vi "Make.vi"(8 "error in (no error)":errorcluster, 9 "Item Refnum":refnum<vi>, 10 "Target":refnum<vi>, 11 "Abstract Message Rescripter":refnum<class "Abstract Message Rescripter.lvclass">) -> (0 "error out":errorcluster, 3 "Abstract Message Rescripter out":refnum<class "Abstract Message Rescripter.lvclass">)   [LabVIEW 2020, in "Message Rescripter.lvlib" / "Abstract Message Rescripter.lvclass"]
uses:
  Abstract Message Rescripter.lvclass
  MessageMakerProvider/_Message Maker/_Maker Classes/Message Scripter/Message Scripter.lvclass
  MessageMakerProvider/_Message Maker/_Maker Classes/Concrete Send Builder/Concrete Send Builder.lvclass
  Message Rescripter.lvlib
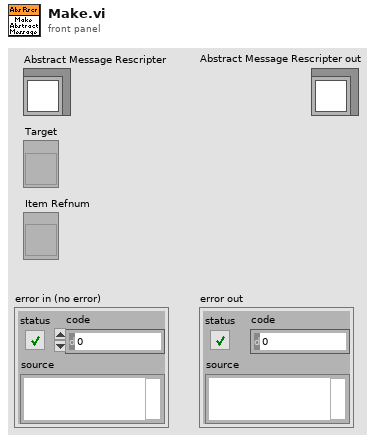
[diagram p1: front panel]
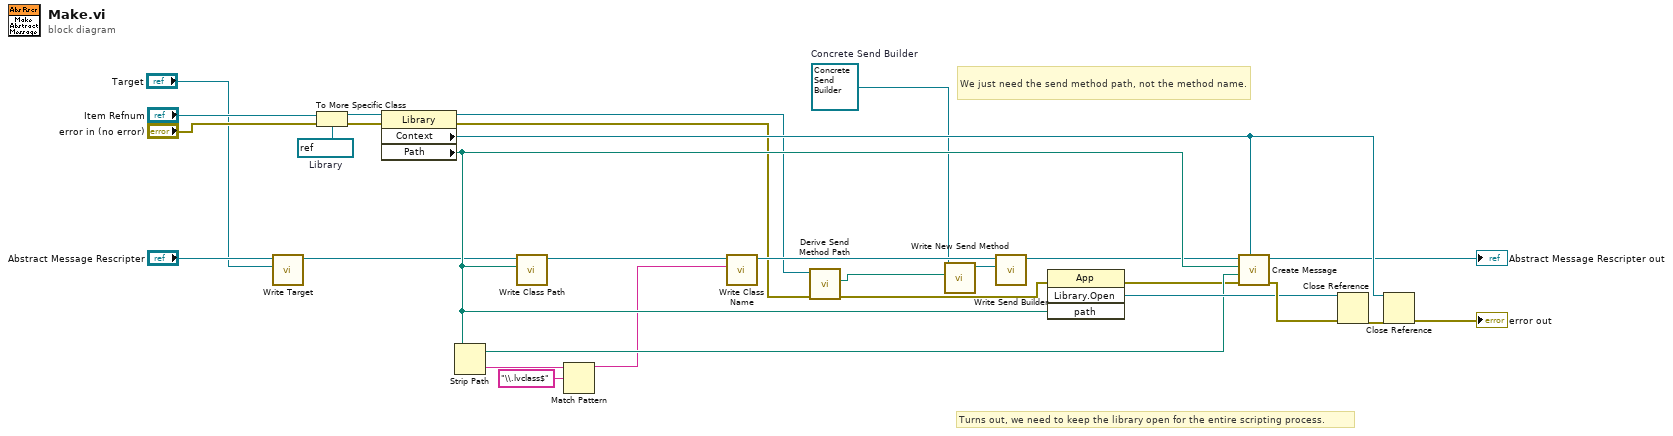
[diagram p0: block diagram]
diagram:
  w27 = refnum<vi> refnum  # Library
  w7 = refnum<class "Concrete Send Builder.lvclass"> refnum  # Concrete Send Builder
  # "We just need the send method path, not the method name."
  # "Turns out, we need to keep the library open for the entire scripting process."
  n1 = call "Write Target.vi"("Target"="Target", "Message Scripter in"="Abstract Message Rescripter") -> ("Message Scripter out"=w2:refnum<class "Abstract Message Rescripter.lvclass">)  [unwired: 9 in]
  n2 = To More Specific Class(target class=w27, reference="Item Refnum", error in="error in (no error)") -> (specific class reference=w25:refnum<vi>, error out=w26:errorcluster)
  n3 = property class="Library"(reference=w25, error in=w26) -> (reference out=w6:refnum<vi>, error out=w5:errorcluster, "Context"=w28:refnum<vi>, "Path"=w29:path)
  n4 = Strip Path(path=w29) -> (stripped path=w18:path, name=w10:string)
  n5 = call "Write Class Path.vi"("Class Path"=w29, "Message Scripter in"=w2) -> ("Message Scripter out"=w17:refnum<class "Abstract Message Rescripter.lvclass">)  [unwired: 9 in]
  n6 = Match Pattern(string=w10, regular expression="\\.lvclass$") -> (before substring=w8:string)  [unwired: 1 in, 3 out]
  n7 = call "Write Class Name.vi"("Class Name"=w8, "Message Scripter in"=w17) -> ("Message Scripter out"=w9:refnum<class "Abstract Message Rescripter.lvclass">)  [unwired: 9 in]
  n8 = call "Derive Send Method Path.vi"("error in (no error)"=w5, "Library"=w6) -> ("error out"=w4:errorcluster, "Send VI Path"=w21:path)  [unwired: 7 in, 1 out]
  n9 = call "Write New Send Method.vi"("New Send Method"=w21, "Concrete Send Builder in"=w7) -> ("Concrete Send Builder out"=w19:refnum<class "Concrete Send Builder.lvclass">)  [unwired: 9 in]
  n10 = call "Write Send Builder.vi"("Message Maker.lvlib:Send Builder.lvclass"=w19, "Message Scripter in"=w9) -> ("Message Scripter out"=w20:refnum<class "Abstract Message Rescripter.lvclass">)  [unwired: 9 in]
  n11 = invoke class="App" method="Library.Open"(error in=w4, "path"=w29) -> (error out=w12:errorcluster, "Open Library"=w22:refnum<vi>)  [unwired: 2 in, 2 out]
  n12 = call "Create Message.vi"("AppInst"=w28, "error in (no error)"=w12, "Destination Path"=w18, "Actor class path"=w29, "Message Maker in"=w20) -> ("error out"=w23:errorcluster, "Message Maker out"=→"Abstract Message Rescripter out":refnum<class "Abstract Message Rescripter.lvclass">)  [unwired: 5 in]
  n13 = Close Reference(reference=w22, error in (no error)=w23) -> (error out=w24:errorcluster)
  n14 = Close Reference(reference=w28, error in (no error)=w24) -> (error out=→"error out":errorcluster)
